vi "MakePaths.vi"(0 "File path":path, 1 "File name index":dbl) -> (2 ".avi-file path":path, 3 ".bin-file path":path, 4 ".tdms-file path":path)   [LabVIEW 2015]
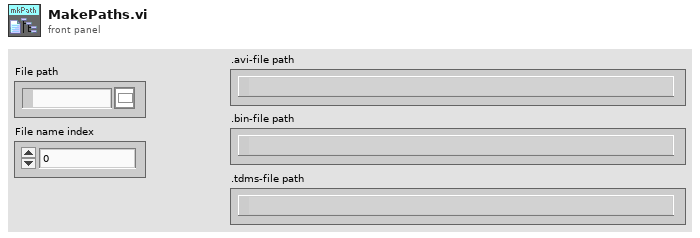
[diagram p1: front panel]
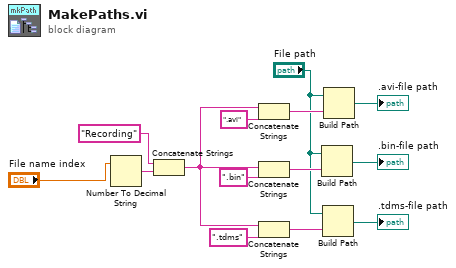
[diagram p0: block diagram]
diagram:
  n1 = Number To Decimal String(number="File name index") -> (decimal integer string=w10:string)  [unwired: 1 in]
  n2 = Concatenate Strings("Recording" ("string"), w10) -> (w5:string)
  n3 = Concatenate Strings(w5, ".avi" ("string")) -> (w8:string)
  n4 = Concatenate Strings(w5, ".bin" ("string")) -> (w7:string)
  n5 = Concatenate Strings(w5, ".tdms" ("string")) -> (w6:string)
  n6 = Build Path(base path="File path", name or relative path=w7) -> (appended path=→".bin-file path":path)
  n7 = Build Path(base path="File path", name or relative path=w6) -> (appended path=→".tdms-file path":path)
  n8 = Build Path(base path="File path", name or relative path=w8) -> (appended path=→".avi-file path":path)
